vi "EncoderTestingDriveDistance.vi"(11 "Distance":dbl) -> ()   [LabVIEW 2015]
uses:
  <vilib>/Rock Robotics/Network Tables/NT Read Number.vi
  <vilib>/addons/control/pid/pid.llb/PID (DBL).vi
  <vilib>/addons/control/pid/NI_PID_pid.lvlib
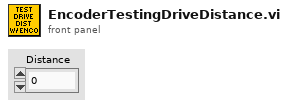
[diagram p1: front panel]
types:
  T1 = typedef "WPI_EncoderDevRef.ctl" = cluster{"DevStatus":errorcluster, "EncoderIndex":T2, "CounterIndex":T3, "DistancePerCount":dbl, "Decoding Type":T4}
  T2 = typedef "FPGA_EncoderIdx.ctl" = enum8{"Enc 0", "Enc 1", "Enc 2", "Enc 3", "Enc 4", "Enc 5", "Enc 6", "Enc 7", "Invalid"}
  T3 = typedef "FPGA_CounterCtrSystemIndex.ctl" = enum8{"Ctr 0", "Ctr 1", "Ctr 2", "Ctr 3", "Ctr 4", "Ctr 5", "Ctr 6", "Ctr 7", "Invalid"}
  T4 = typedef "WPI_EncoderType.ctl" = enum16{"1x", "2x", "4x"}
  T5 = cluster{"proportional gain (Kc)":dbl, "integral time (Ti, min)":dbl, "derivative time (Td, min)":dbl}
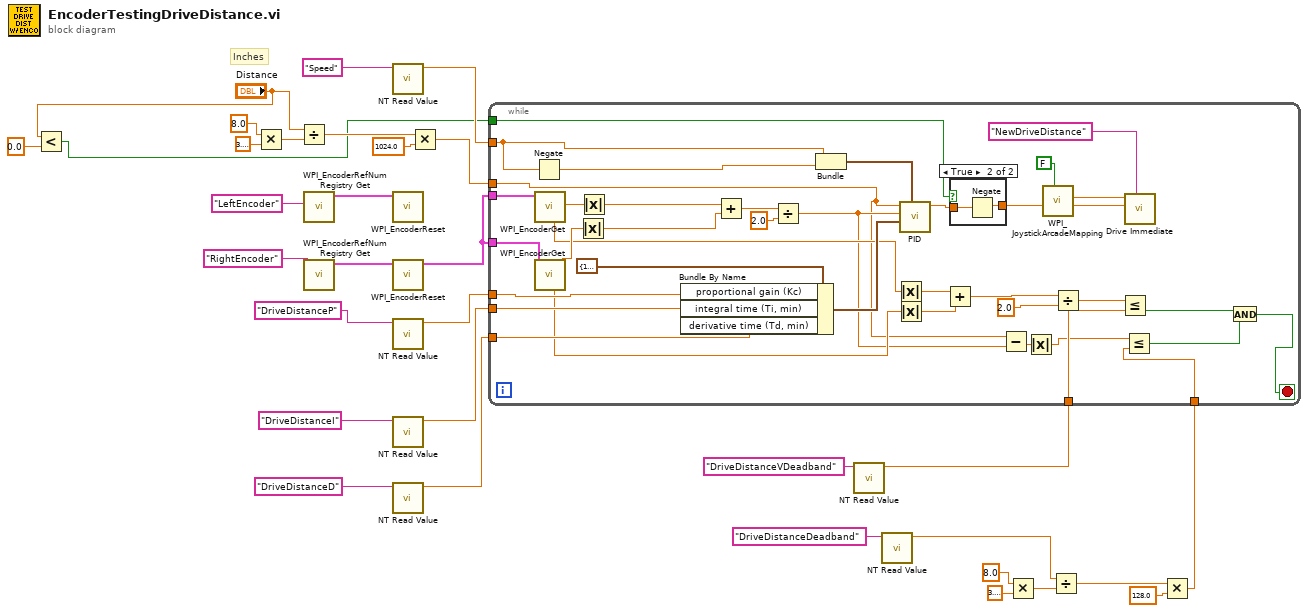
[diagram p0: block diagram]
diagram:
  # "Inches"
  n1 = Less?(x="Distance", y=0.0) -> (x < y?=w1:bool)
  n2 = Multiply(x=8.0, y=3.141592653589793) -> (x*y=w26:dbl)
  n3 = Divide(x="Distance", y=w26) -> (x/y=w25:dbl)
  n4 = call <vilib>:"WPI_EncoderRefNum Registry Get.vi"("refnum name"="LeftEncoder") -> ("EncoderDevRef"=w32:T1)  [unwired: 9 in, 1 out]
  n5 = call <vilib>:"WPI_EncoderRefNum Registry Get.vi"("refnum name"="RightEncoder") -> ("EncoderDevRef"=w31:T1)  [unwired: 9 in, 1 out]
  n6 = call-poly <vilib>:"NT Read Value.vi"("Name"="Speed") -> ("Numeric"=w21:dbl)  [unwired: 9 in, 1 out]
  n7 = call <vilib>:"WPI_EncoderReset.vi"("EncoderDevRef"=w32) -> ()  [unwired: 9 in, 2 out]
  n8 = call <vilib>:"WPI_EncoderReset.vi"("EncoderDevRef"=w31) -> ("EncoderDevRef"=w11:T1)  [unwired: 9 in, 1 out]
  n9 = call-poly <vilib>:"NT Read Value.vi"("Name"="DriveDistanceP") -> ("Numeric"=w16:dbl)  [unwired: 9 in, 1 out]
  n10 = call-poly <vilib>:"NT Read Value.vi"("Name"="DriveDistanceI") -> ("Numeric"=w15:dbl)  [unwired: 9 in, 1 out]
  n11 = call-poly <vilib>:"NT Read Value.vi"("Name"="DriveDistanceD") -> ("Numeric"=w14:dbl)  [unwired: 9 in, 1 out]
  n12 = Multiply(x=w25, y=1024.0) -> (x*y=w20:dbl)
  n13 = call-poly <vilib>:"NT Read Value.vi"("Name"="DriveDistanceVDeadband") -> ("Numeric"=w12:dbl)  [unwired: 9 in, 1 out]
  n14 = call-poly <vilib>:"NT Read Value.vi"("Name"="DriveDistanceDeadband") -> ("Numeric"=w5:dbl)  [unwired: 9 in, 1 out]
  n15 = Multiply(x=8.0, y=3.141592653589793) -> (x*y=w8:dbl)
  n16 = Divide(x=w5, y=w8) -> (x/y=w7:dbl)
  n17 = Multiply(x=w7, y=128.0) -> (x*y=w4:dbl)
  n18 = while {
    tunnel: w11 -> [w71]
    tunnel: w11 -> [w70]
    tunnel: w21 -> [w65]
    tunnel: w20 -> [w40]
    tunnel: w16 -> [w62]
    tunnel: w15 -> [w61]
    tunnel: w14 -> [w60]
    tunnel: w12 -> [w46]
    tunnel: w4 -> [w42]
    tunnel: w1 -> [w33]
    stop <- w45 stop-if-true
    n19 = Negate(x=w65) -> (-x=w66:dbl)
    n20 = call <vilib>:"WPI_EncoderGet.vi"("EncoderDevRef"=w71) -> ("Distance"=w54:dbl, "Rate"=w48:dbl)  [unwired: 5 in, 4 out]
    n21 = call <vilib>:"WPI_EncoderGet.vi"("EncoderDevRef"=w70) -> ("Distance"=w69:dbl, "Rate"=w49:dbl)  [unwired: 5 in, 4 out]
    n22 = Absolute Value(x=w69) -> (abs(x)=w36:dbl)
    n23 = Absolute Value(x=w54) -> (abs(x)=w37:dbl)
    n24 = Bundle By Name(cluster=T5 {"proportional gain (Kc)"=1.0, "integral time (Ti, min)"=0.01, "derivative time (Td, min)"=0.0} ("PID gains"), "proportional gain (Kc)"=w62, "integral time (Ti, min)"=w61, "derivative time (Td, min)"=w60) -> (w59:T5)
    n25 = Add(x=w37, y=w36) -> (x+y=w68:dbl)
    n26 = Divide(x=w68, y=2.0) -> (x/y=w41:dbl)
    n27 = Bundle("Numeric"=w65, w66) -> (w64:cluster{"Numeric":dbl, dbl})  [unwired: 1 in]
    n28 = Absolute Value(x=w48) -> (abs(x)=w51:dbl)
    n29 = Absolute Value(x=w49) -> (abs(x)=w50:dbl)
    n30 = call-poly <vilib>:"PID.vi"("output range"=w64, "PID gains"=w59, "process variable"=w41, "setpoint"=w40) -> ("output"=w35:dbl)  [unwired: 6 in, 1 out]
    n31 = Add(x=w51, y=w50) -> (x+y=w53:dbl)
    n32 = case shown="True" w33 {
      tunnel: w35 -> [w72 w73]
      tunnel: [w72 w74] -> w34
      frame False {
      }
      frame True {
        n33 = Negate(x=w73) -> (-x=w74:dbl)
      }
    }
    n34 = Subtract(x=w40, y=w41) -> (x-y=w39:dbl)
    n35 = Absolute Value(x=w39) -> (abs(x)=w38:dbl)
    n36 = call <vilib>:"WPI_JoystickArcadeMapping.vi"("Square Inputs"=FALSE, "Y axis value"=w34) -> ("Right Motor Value"=w57:dbl, "Left Motor Value"=w56:dbl)  [unwired: 8 in]
    n37 = Divide(x=w53, y=2.0) -> (x/y=w47:dbl)
    n38 = Less Or Equal?(x=w47, y=w46) -> (x <= y?=w44:bool)
    n39 = Less Or Equal?(x=w38, y=w42) -> (x <= y?=w43:bool)
    n40 = call "Drive Immediate.vi"("Description"="NewDriveDistance", "Right Setpoint"=w57, "Left Setpoint"=w56) -> ()  [unwired: 8 in, 1 out]
    n41 = And(x=w44, y=w43) -> (x .and. y?=w45:bool)
  }
